vi "Factorial_FormulaNode.vi"() -> ()   [LabVIEW 2022 SP3]
panel:
  in  "stop":bool
  out "fact":dbl
  in  "n":dbl
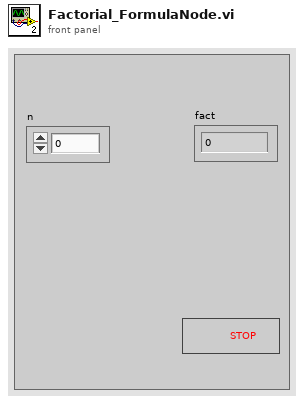
[diagram p1: front panel]
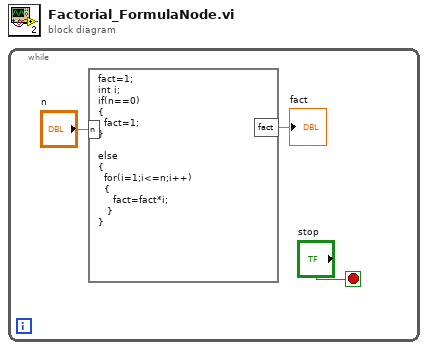
[diagram p0: block diagram]
diagram:
  n1 = while {
    stop <- "stop" stop-if-true
    n2 = formula code="fact=1;\nint i;\nif(n==0)\n{\n  fact=1;\n}\n\nelse\n{\n  for(i=1;i<=n;i++)\n  {\n     fact=fact*i;\n   }\n}"("n"="n") -> ("fact"=→"fact":dbl)
  }
